vi "1.3.2-Serial Write.vi"(0 "Transmit":refnum<k21>="Port8/DIO0", 1 "Write FIFO":refnum<k21>="Write FIFO", 7 "baud rate (9600)":u32=9600, 9 "data bits (8)":i32=8 min=5 max=8 step=1, 11 "parity (0:none)":enum16{"None", "Odd", "Even", "Mark", "Space"}(ring), 12 "stop bits (10: 1 bit)":u16(ring)=10 items=["1.0"=10, "1.5"=15, "2.0"=20], 13 "Invert Polarity?":bool) -> ()   [LabVIEW 2010]
uses:
  <vilib>/eio/EIONode/EIONode.xnode
  <vilib>/eio/EIOMethodNode/EIOMethodNode.xnode
  <vilib>/rvi/DataTransferAndStorage/Container/XNode/niFpgaContainer.xnode
  <vilib>/rvi/DataTransferAndStorage/Container/Common/niFpgaContainerMethod.ctl
  <vilib>/rvi/FIFO/Fifo_Types/niFpgaFifoControlLogicControl.ctl
  <vilib>/rvi/DataTransferAndStorage/Container/Common/niFpgaContainerMetaDataKey.ctl
  <vilib>/rvi/DataTransferAndStorage/Container/Common/niFpgaContainerExecOnDevCompGetState.vi
  <vilib>/rvi/FIFO/Fifo_Resource/nirvififoEmulationSetSize.vi
  <vilib>/rvi/DataTransferAndStorage/Container/Common/niFpgaContainerGetUniqueNameForEmu.vi
  <vilib>/rvi/eio/common/nirviEmuReportErrorAndStop.vi
  <vilib>/rvi/DataTransferAndStorage/Container/Common/niFpgaTransferTypeControl.ctl
  <vilib>/rvi/interface/RandomDataEmulation/nirviRandomDataFPGAFIFO.vi
  <vilib>/rvi/interface/RandomDataEmulation/niFpgaRandomDataHandleErrors.vi
  <vilib>/rvi/DataTransferAndStorage/FIFO/niFpgaPeerToPeerStreamState.ctl
  1.0-Hindbrain Global.vi
panel:
  out "Read: Transmission Error":bool
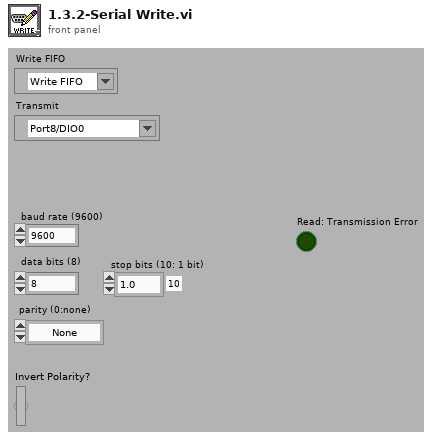
[diagram p1: front panel]
types:
  T1 = typedef "niFpgaFifoControlLogicControl.ctl" = enum16{"Slice Fabric", "Target Optimal", "Built-in"}
  T2 = typedef "niFpgaContainerMethod.ctl" = enum16{"<none>", "write", "read", "clear", "getNumberOfElementsToWrite", "getNumberOfElementsToRead", "enable", "disable", "flushAndDisable", "getStreamState", "readA", "readB", "dramWrite", "dramWriteWithByteEnables", "dramRequestData", "dramRetrieveData"}
  T3 = typedef "niFpgaTransferTypeControl.ctl" = enum16{"Target-Scoped", "Host to Target - DMA", "Target to Host - DMA", "Peer to Peer Reader", "Peer to Peer Writer", "Bidirectional"}
  T4 = typedef "niFpgaPeerToPeerStreamState.ctl" = enum16{"Unlinked", "Disabled", "Enabled", "Flushing"}
  T5 = typedef "niFpgaContainerMetaDataKey.ctl" = enum16{"FPGA FIFO", "FPGA Memory", "FPGA Register"}
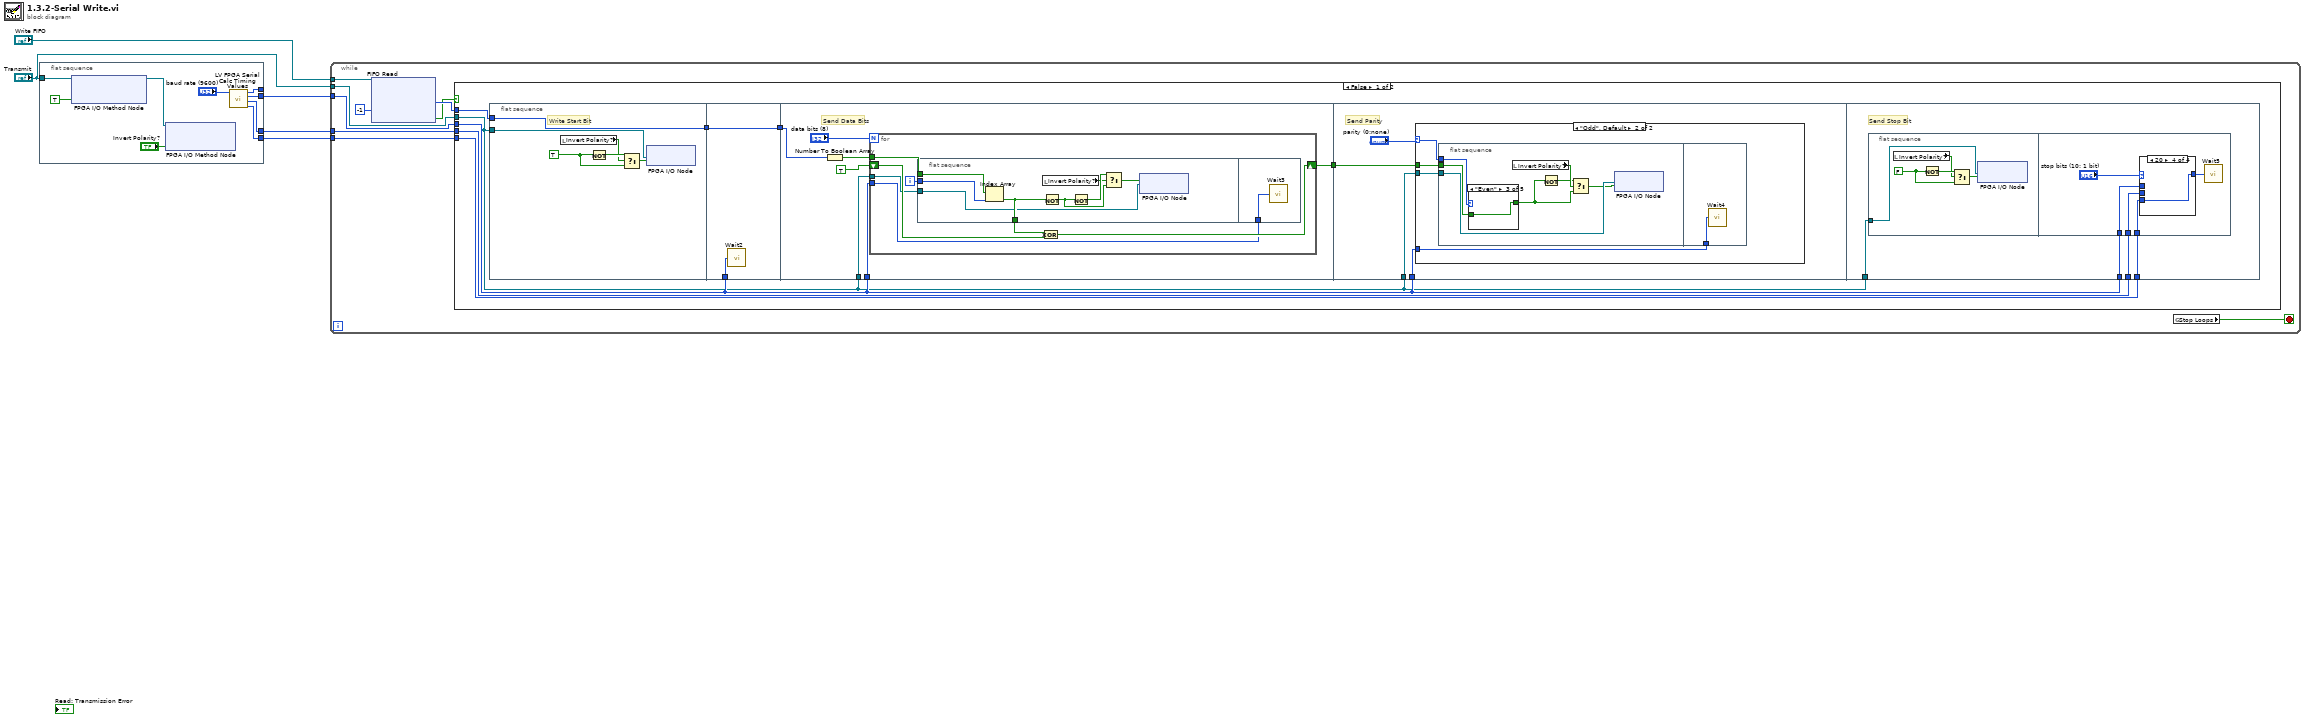
[diagram p0: block diagram]
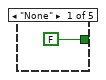
[diagram p3: hidden frame]
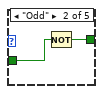
[diagram p4: hidden frame]
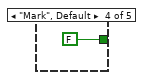
[diagram p5: hidden frame]
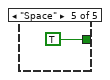
[diagram p6: hidden frame]
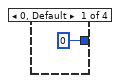
[diagram p7: hidden frame]
diagram:
  n1 = flat-sequence {
    tunnel: [w10] -> w5
    tunnel: [w13] -> _
    tunnel: [w12] -> w4
    tunnel: [w11] -> w3
    tunnel: "Transmit" -> [w8]
    frame #0 {
      n2 = xnode "FPGA I/O Method Node"("FPGA I/O In"=w8, "Enable"=TRUE ("Digital Enable")) -> ("FPGA I/O Out"=w7:refnum<k21>)
      n3 = xnode "FPGA I/O Method Node"("FPGA I/O In"=w7, "Data"="Invert Polarity?") -> ()  [unwired: 1 out]
      n4 = call "LV FPGA Serial Calc Timing Values.vi"("baud rate (1000000)"="baud rate (9600)") -> ("Two Bit"=w11:u32, "One and Half Bit"=w12:u32, "One Bit"=w10:u32, "Half Bit"=w13:u32)  [unwired: 1 in, 2 out]
    }
  }
  n5 = while {
    tunnel: w3 -> [w23]
    tunnel: w4 -> [w22]
    tunnel: w5 -> [w21]
    tunnel: "Transmit" -> [w20]
    tunnel: "Write FIFO" -> [w16]
    stop <- w15 stop-if-true
    n6 = xnode ("FIFO Read")("Timeout"=-1, "FIFO In"=w16) -> ("Element"=w19:u8, "Timed Out?"=w17:bool)  [unwired: 1 out]
    n7 = case shown="False" w17 {
      tunnel: w23 -> [w345 _]
      tunnel: w22 -> [w344 _]
      tunnel: w21 -> [w343 _]
      tunnel: w20 -> [w342 _]
      tunnel: w19 -> [w341 _]
      frame False {
        n8 = flat-sequence {
          tunnel: w342 -> [w354]
          tunnel: w341 -> [w349]
          tunnel: [w349] -> w348
          tunnel: w343 -> [w356]
          tunnel: [w355] -> w347
          tunnel: w348 -> [w355]
          tunnel: w343 -> [w363]
          tunnel: [w361] -> w346
          tunnel: w342 -> [w359]
          tunnel: w347 -> [w358]
          tunnel: w343 -> [w382]
          tunnel: w346 -> [w383]
          tunnel: w342 -> [w381]
          tunnel: w343 -> [w405]
          tunnel: w344 -> [w404]
          tunnel: w345 -> [w403]
          tunnel: w342 -> [w402]
          frame #0 {
            w352 = TRUE
            # "Write Start Bit"
            n9 = local read "Invert Polarity?"() -> (w351:bool)
            n10 = Not(x=w352) -> (.not. x?=w353:bool)
            n11 = Select(t=w353, s=w351, f=w352) -> (s? t:f=w350:bool)
            n12 = xnode "FPGA I/O Node"("I/O Item"=w350, "FPGA I/O In"=w354) -> ()  [unwired: 1 out]
          }
          frame #1 {
            n13 = call "Wait2"("Count(Ticks)"=w356) -> ()  [unwired: 1 out]
          }
          frame #2 {
            # "Send Data Bits"
            n14 = Number To Boolean Array(number=w358) -> (Boolean array=w360:bool[])
            n15 = for {
              N: "data bits (8)" -> [_]
              tunnel: w363 -> [w367]
              shift-right: [w370] -> w361
              shift-left: TRUE -> [w369]
              tunnel: w360 -> [w366]
              tunnel: w359 -> [w364]
              i -> [w368]
              n16 = flat-sequence {
                tunnel: w368 -> [w378]
                tunnel: w366 -> [w377]
                tunnel: [w376] -> w365
                tunnel: w364 -> [w375]
                tunnel: w367 -> [w379]
                frame #0 {
                  n17 = Index Array(array=w377, index=w378) -> (element=w376:bool)
                  n18 = local read "Invert Polarity?"() -> (w372:bool)
                  n19 = Not(x=w376) -> (.not. x?=w373:bool)
                  n20 = Not(x=w373) -> (.not. x?=w374:bool)
                  n21 = Select(t=w374, s=w372, f=w373) -> (s? t:f=w371:bool)
                  n22 = xnode "FPGA I/O Node"("I/O Item"=w371, "FPGA I/O In"=w375) -> ()  [unwired: 1 out]
                }
                frame #1 {
                  n23 = call "Wait3"("Count(Ticks)"=w379) -> ()  [unwired: 1 out]
                }
              }
              n24 = Exclusive Or(1:w369, 2:w365) -> (0:w370:bool)
            }
          }
          frame #3 {
            # "Send Parity"
            n25 = case shown="\"Odd\", Default" "parity (0:none)" {
              selector: "parity (0:none)" -> [_ w387]
              tunnel: w383 -> [_ w386]
              tunnel: w382 -> [_ w385]
              tunnel: w381 -> [_ w384]
              frame "None" {
              }
              frame "Odd", Default {
                n26 = flat-sequence {
                  tunnel: w386 -> [w393]
                  tunnel: w387 -> [w394]
                  tunnel: w384 -> [w392]
                  tunnel: w385 -> [w401]
                  frame #0 {
                    n27 = case shown="\"Even\"" w394 {
                      tunnel: w393 -> [_ w397 w398 _ _]
                      tunnel: [FALSE ("y") w396 w398 FALSE ("y") TRUE ("y")] -> w389
                      frame "None" {
                      }
                      frame "Odd" {
                        n28 = Not(x=w397) -> (.not. x?=w396:bool)
                      }
                      frame "Even" {
                      }
                      frame "Mark", Default {
                      }
                      frame "Space" {
                      }
                    }
                    n29 = local read "Invert Polarity?"() -> (w391:bool)
                    n30 = Not(x=w389) -> (.not. x?=w390:bool)
                    n31 = Select(t=w390, s=w391, f=w389) -> (s? t:f=w388:bool)
                    n32 = xnode "FPGA I/O Node"("I/O Item"=w388, "FPGA I/O In"=w392) -> ()  [unwired: 1 out]
                  }
                  frame #1 {
                    n33 = call "Wait4"("Count(Ticks)"=w401) -> ()  [unwired: 1 out]
                  }
                }
              }
            }
          }
          frame #4 {
            # "Send Stop Bit"
            n34 = flat-sequence {
              tunnel: w402 -> [w410]
              tunnel: w405 -> [w415]
              tunnel: w404 -> [w414]
              tunnel: w403 -> [w413]
              frame #0 {
                w408 = FALSE
                n35 = local read "Invert Polarity?"() -> (w407:bool)
                n36 = Not(x=w408) -> (.not. x?=w409:bool)
                n37 = Select(t=w409, s=w407, f=w408) -> (s? t:f=w406:bool)
                n38 = xnode "FPGA I/O Node"("I/O Item"=w406, "FPGA I/O In"=w410) -> ()  [unwired: 1 out]
              }
              frame #1 {
                n39 = case shown="20" "stop bits (10: 1 bit)" {
                  tunnel: w415 -> [_ w417 _ _]
                  tunnel: w414 -> [_ _ w418 _]
                  tunnel: w413 -> [_ _ _ w419]
                  tunnel: [u32 0 ("One Bit") w417 w418 w419] -> w412
                  frame 0, Default {
                  }
                  frame 10 {
                  }
                  frame 15 {
                  }
                  frame 20 {
                  }
                }
                n40 = call "Wait5"("Count(Ticks)"=w412) -> ()  [unwired: 1 out]
              }
            }
          }
        }
      }
      frame True {
      }
    }
    n41 = global read "1.0-Hindbrain Global.vi" "Stop Loops"() -> (w15:bool)
  }
